vi "Main.vi"(11 "Module Admin":refnum<class "Delacor_lib_QMH_Cloneable Module Admin.lvclass">) -> ()   [LabVIEW 2025, in "USB IO.lvlib"]
doc: "This template is based off of the Queued Message Handler design pattern and the Queued Message Handler project template that ships with LabVIEW.\n\nThe main difference is that the queue is private to this module and communication between modules is performed via Broadcast and Request events.\n\nRequest events are wrapped in public API methods and are handled in the Event Handling Loop (EHL) of this VI. Any module can register for Broadcast events sent by this module. The EHL generates messages based on user interface actions.\n\nThe Message Handling Loop (MHL) processes messages generated by the EHL, or by other messages. The messages are string values, so new messages can be added easily to the Message Cases case structure in the MHL. Each message cluster can also provide an optional value for Message Data, which is a variant that can be converted to whatever message-specific data is required.\n_____\nBased on DQMH Dev Tools: Project Template 7.1.2.1547."
uses:
  USB IO.lvlib
  <vilib>/Delacor/Delacor QMH/Libraries/Message Queue_class/Delacor_lib_QMH_Message Queue.lvclass/Delacor_lib_QMH_Message Queue.ctl
  <vilib>/Delacor/Delacor QMH/Libraries/Cloneable Module Admin_class/Delacor_lib_QMH_Cloneable Module Admin.lvclass/Delacor_lib_QMH_Cloneable Module Admin.ctl
  <vilib>/Delacor/Delacor QMH/Libraries/Module Admin_class/Delacor_lib_QMH_Module Admin.lvclass/Delacor_lib_QMH_Module Admin.ctl
  <vilib>/Delacor/Delacor QMH/Libraries/Message Queue_class/Delacor_lib_QMH_Message Queue.lvclass
  Module Data--cluster.ctl
  <vilib>/Utility/miscctls.llb/LVPointTypeDef.ctl
  <vilib>/Delacor/Delacor QMH/Libraries/Message Queue_class/Delacor_lib_QMH_Enqueue Message (Single).vi
  Stop Argument--cluster.ctl
  <vilib>/Delacor/Delacor QMH/Libraries/Cloneable Module Admin_class/Delacor_lib_QMH_Cloneable Module Admin.lvclass
  Display Lines (Reply Payload)--cluster.ctl
  Display Lines Argument--cluster.ctl
  Classes/USB IO generic/USB IO.lvclass
  select child (Reply Payload)--cluster.ctl
  Classes/Hardware Selection.ctl
  select child Argument--cluster.ctl
  Classes/Arduino Uno/Arduino Uno.lvclass
  Classes/USB-6000/USB-6000.lvclass
  read config (Reply Payload)--cluster.ctl
  read config Argument--cluster.ctl
  init device (Reply Payload)--cluster.ctl
  init device Argument--cluster.ctl
  stop device (Reply Payload)--cluster.ctl
  stop device Argument--cluster.ctl
  C:/Users/grove/Desktop/LabVIEW/Git/dqmh-lvoop-template/Libraries/USB IO/Classes/USB IO generic/USB IO.lvclass
  C:/Users/grove/Desktop/LabVIEW/Git/dqmh-lvoop-template/Libraries/USB IO/Classes/USB-6000/USB-6000.lvclass
  C:/Users/grove/Desktop/LabVIEW/Git/dqmh-lvoop-template/Libraries/USB IO/Classes/Arduino Uno/Arduino Uno.lvclass
panel:
  out "error out":errorcluster
  out "Status":string
  in  "Simulate EHL Error":bool
  in  "Simulate MHL Error":bool
  # "Other processes communicate with this Module via its Public API (wrappers for its Request Events).\n\nThis Module communicates with other processes via its Broadcast Events.\nAny process that wants to receive these messages can register for this module's Broadcast events."
  # "This template is for the DQMH framework. See the block diagram for more information on how to use this template."
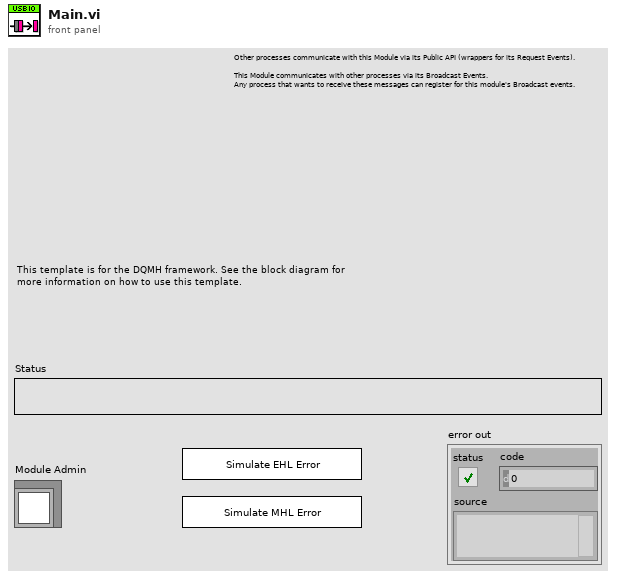
[diagram p1: front panel]
types:
  T1 = typedef "USB IO.lvlib/Request Events--cluster.ctl" = cluster{"Stop Module":refnum<user-event>, "Show Panel":refnum<user-event>, "Hide Panel":refnum<user-event>, "Show Diagram":refnum<user-event>, "Get Module Execution Status":refnum<user-event>, "Display Lines":refnum<user-event>, "select child":refnum<user-event>, "read config":refnum<user-event>, "init":refnum<user-event>, "init device":refnum<user-event>, "stop device":refnum<user-event>}
  T2 = typedef "USB IO.lvlib/Module Data--cluster.ctl" = cluster{"Status":string, "USB IO.lvlib:USB IO.lvclass":refnum<class "USB IO.lvclass">}
  T3 = enum32{"invalid lock state", "Not Locked", "Locked (No Password)", "Password-protected"}
  T4 = typedef "USB IO.lvlib/Stop Argument--cluster.ctl" = cluster{"Module ID":i32, "Origin":string, "Exit via Stop Module Req?":bool, "Wait for Module to stop?":bool}
  T5 = typedef "USB IO.lvlib/Display Lines Argument--cluster.ctl" = cluster{"Module ID":i32, "Wait Notifier":refnum<notifier>, "wait for reply":bool}
  T6 = typedef "USB IO.lvlib/select child Argument--cluster.ctl" = cluster{"Module ID":i32, "Hardware":T7, "Wait Notifier":refnum<notifier>, "wait for reply":bool}
  T7 = typedef "Hardware Selection.ctl" = enum16{"Simulation", "USB-6000", "USB-6001", "Arduino Uno"}
  T8 = typedef "USB IO.lvlib/read config Argument--cluster.ctl" = cluster{"Module ID":i32, "Path":path, "Wait Notifier":refnum<notifier>, "wait for reply":bool}
  T9 = typedef "USB IO.lvlib/init device Argument--cluster.ctl" = cluster{"Module ID":i32, "Variant":variant, "Wait Notifier":refnum<notifier>, "wait for reply":bool}
  T10 = typedef "USB IO.lvlib/stop device Argument--cluster.ctl" = cluster{"Module ID":i32, "Wait Notifier":refnum<notifier>, "wait for reply":bool}
  T11 = typedef "LVPointTypeDef.ctl" = cluster{"Horizontal":i16, "Vertical":i16}
  T12 = enum32{"Invalid", "Standard", "Closed", "Hidden", "Minimized", "Maximized"}
  T13 = typedef "USB IO.lvlib/Display Lines (Reply Payload)--cluster.ctl" = cluster{"Module ID":i32, "Lines":string[], "Values":i32[], "error":errorcluster}
  T14 = typedef "USB IO.lvlib/select child (Reply Payload)--cluster.ctl" = cluster{"Module ID":i32, "error":errorcluster}
  T15 = typedef "USB IO.lvlib/read config (Reply Payload)--cluster.ctl" = cluster{"Module ID":i32, "error":errorcluster}
  T16 = typedef "USB IO.lvlib/init device (Reply Payload)--cluster.ctl" = cluster{"Module ID":i32, "error":errorcluster}
  T17 = typedef "USB IO.lvlib/stop device (Reply Payload)--cluster.ctl" = cluster{"Module ID":i32, "error":errorcluster}
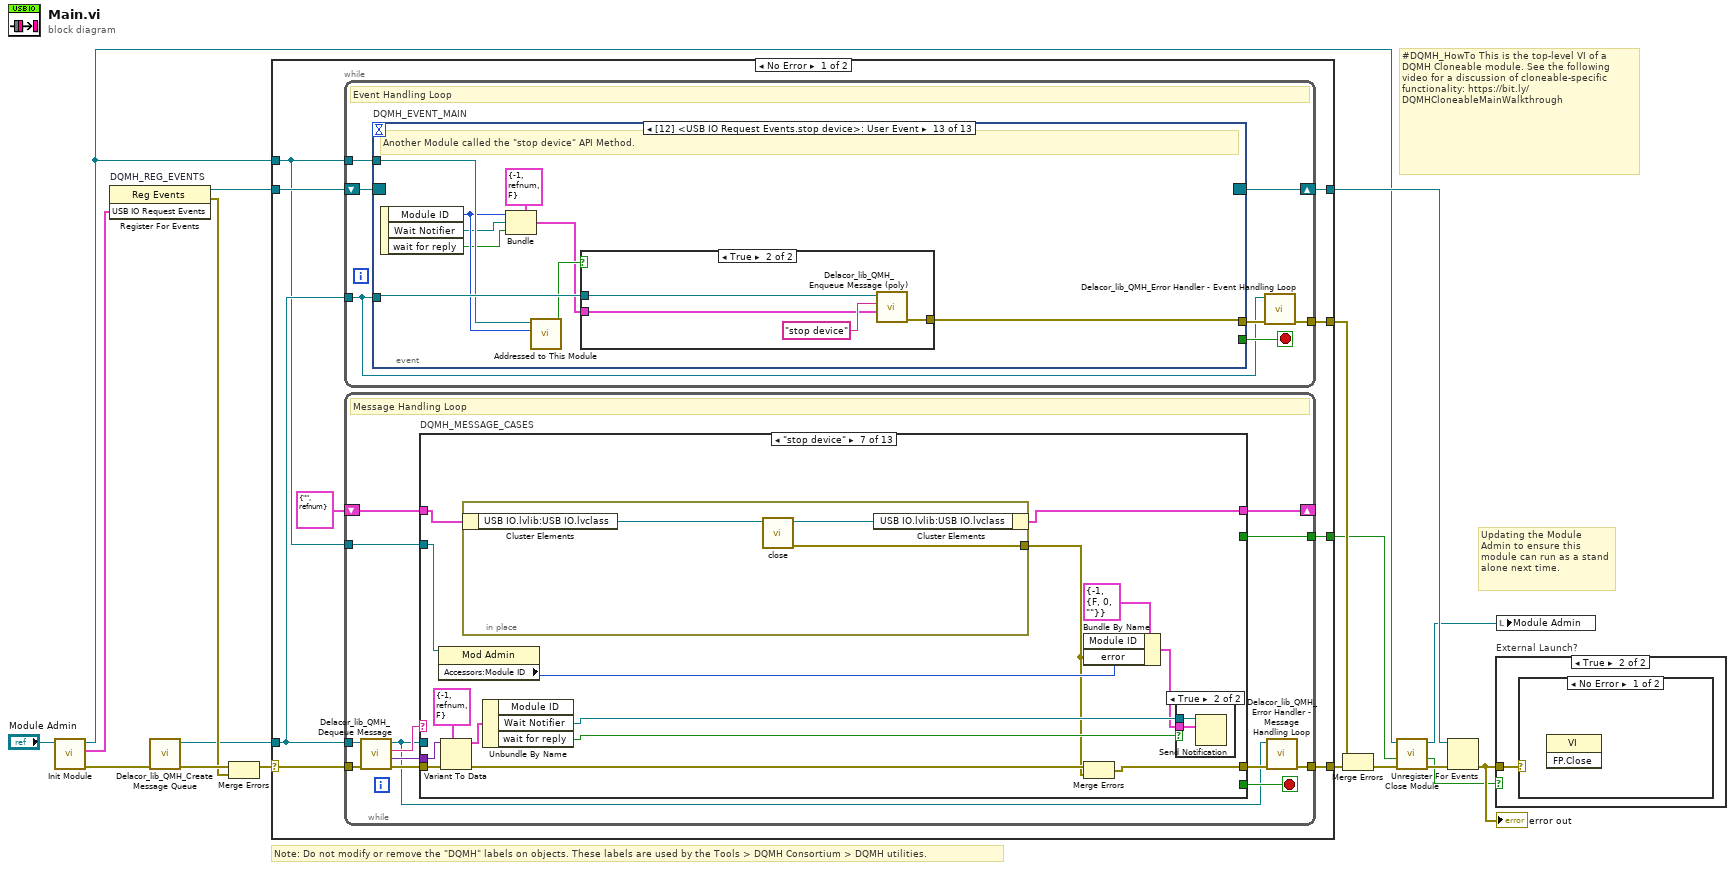
[diagram p0: block diagram]
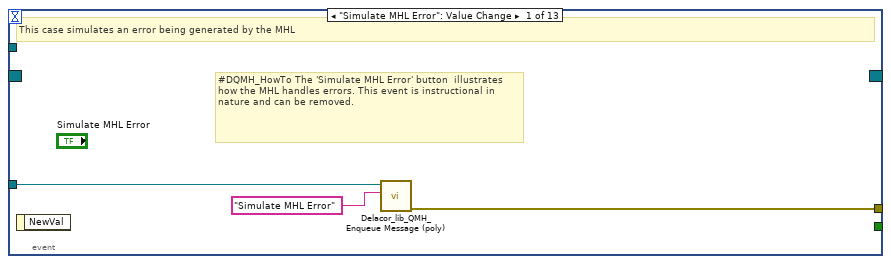
[diagram p2: hidden frame]
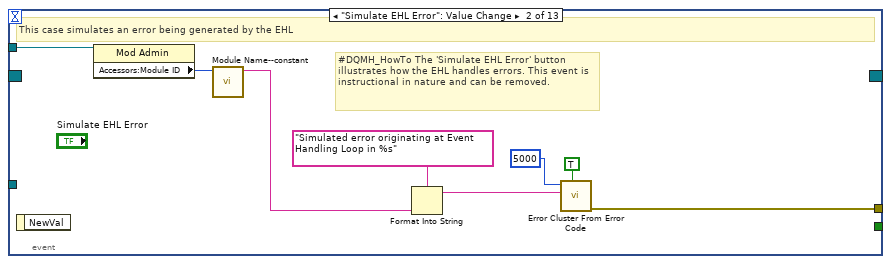
[diagram p3: hidden frame]
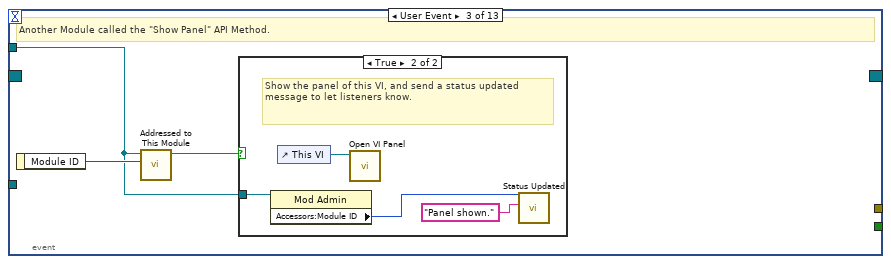
[diagram p4: hidden frame]
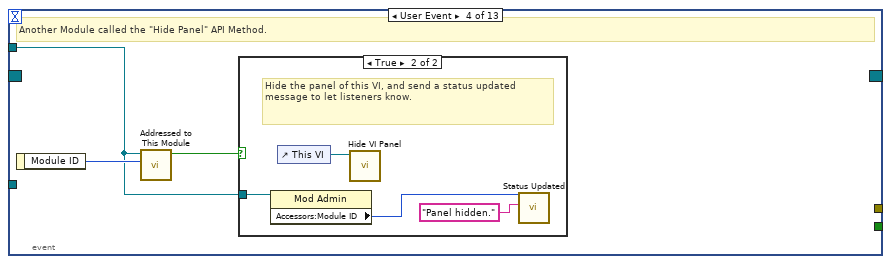
[diagram p6: hidden frame]
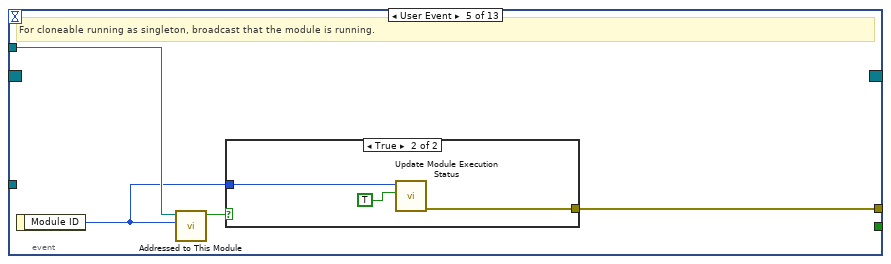
[diagram p8: hidden frame]
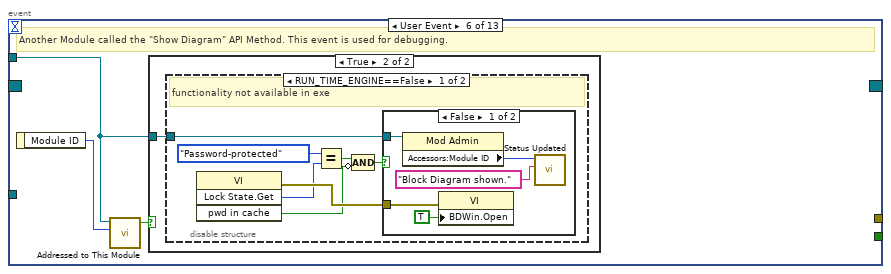
[diagram p10: hidden frame]
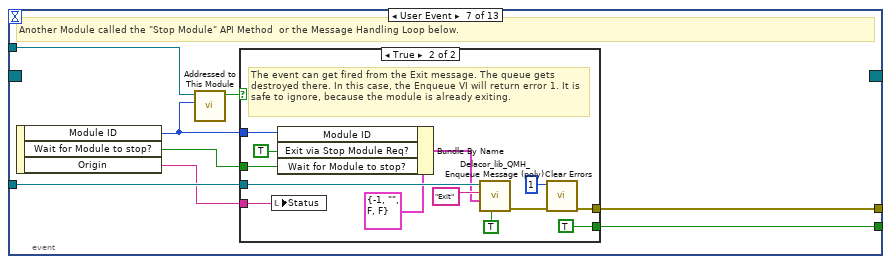
[diagram p14: hidden frame]
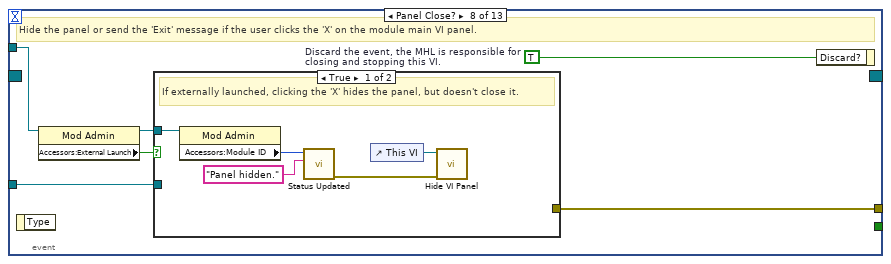
[diagram p16: hidden frame]
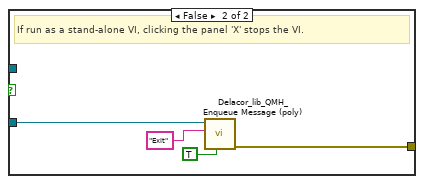
[diagram p17: hidden frame]
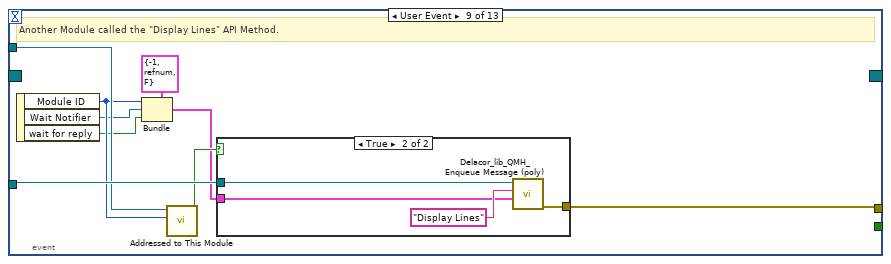
[diagram p18: hidden frame]
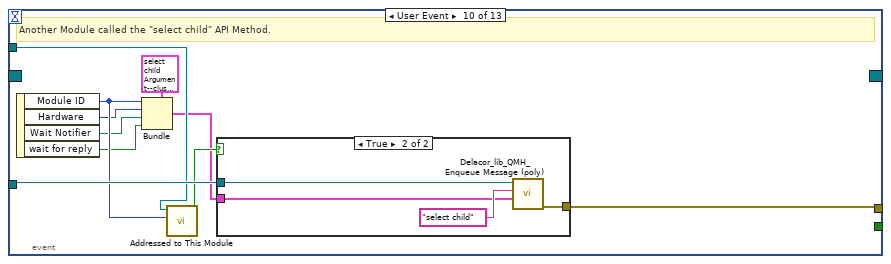
[diagram p20: hidden frame]
diagram:
  # "#DQMH_HowTo This is the top-level VI of a DQMH Cloneable module. See the following video for a discussion of cloneable-specific functionality: https://bit.ly/DQMHCloneableMainWalkthrough"
  # "Note: Do not modify or remove the \"DQMH\" labels on objects. These labels are used by the Tools > DQMH Consortium > DQMH utilities."
  # "Updating the Module Admin to ensure this module can run as a stand alone next time."
  n1 = call "Init Module.vi"("Cloneable Module Admin in"="Module Admin") -> ("error out"=w15:errorcluster, "USB IO Request Events"=w7:T1, "Cloneable Module Admin out"=w4:refnum<class "Delacor_lib_QMH_Cloneable Module Admin.lvclass">)  [unwired: 8 in]
  n2 = register-events "DQMH_REG_EVENTS"(w7) -> (reference out=w8:refnum<event-registration>, error out=w10:errorcluster)  [unwired: 2 in]
  n3 = call <vilib>:"Delacor_lib_QMH_Create Message Queue.vi"("error in"=w15) -> ("error out"=w12:errorcluster, "Message Queue"=w6:refnum<class "Delacor_lib_QMH_Message Queue.lvclass">)  [unwired: 9 in]
  n4 = Merge Errors(w12, w10) -> (w11:errorcluster)
  n5 = case shown="No Error" w11 {
    selector: w11 -> [w25 w404]
    tunnel: [w27 w403] -> w16
    tunnel: [w24 w402] -> w9
    tunnel: w8 -> [w22 w402]
    tunnel: w6 -> [w21 w395]
    tunnel: [w26 _] -> w17
    tunnel: w4 -> [w20 w398]
    tunnel: [w19 _] -> w2
    frame No Error {
      n6 = while {
        tunnel: w21 -> [w28]
        shift-right: [w31] -> w24
        shift-left: w22 -> [w32]
        tunnel: [w33] -> w26
        tunnel: w20 -> [w29]
        stop <- w30 stop-if-true
        # "Event Handling Loop"
        n7 = event "DQMH_EVENT_MAIN" shown="[12] <USB IO Request Events.stop device>: User Event" {
          selector: w32 -> [_ _ _ _ _ _ _ _ _ _ _ _ _]
          dyn-events: [_ _ _ _ _ _ _ _ _ _ _ _ _] -> w31
          timeout: _ -> [_ _ _ _ _ _ _ _ _ _ _ _ _]
          tunnel: [_ _ _ _ _ _ w86 _ _ _ _ _ _] -> w30
          tunnel: w28 -> [w36 _ _ _ _ _ w89 w106 w127 w141 w155 w169 w182]
          tunnel: [w37 w45 _ _ w63 _ w90 w109 w119 w132 w146 w160 w174] -> w34
          tunnel: w29 -> [_ w44 w46 w53 w61 w67 w88 w107 w125 w139 w153 w167 w180]
          event "Simulate MHL Error": Value Change {
            # "#DQMH_HowTo The 'Simulate MHL Error' button  illustrates how the MHL handles errors. This event is instructional in nature and can be removed."
            # "This case simulates an error being generated by the MHL"
            n8 = event-data() -> ()  [unwired: 1 in, 1 out]
            n9 = call-poly <vilib>:"Delacor_lib_QMH_Enqueue Message (poly).vi"("Message"="Simulate MHL Error", "Message Queue in"=w36) -> ("error out"=w37:errorcluster)  [unwired: 8 in, 1 out]
          }
          event "Simulate EHL Error": Value Change {
            # "#DQMH_HowTo The 'Simulate EHL Error' button  illustrates how the EHL handles errors. This event is instructional in nature and can be removed."
            # "This case simulates an error being generated by the EHL"
            n10 = event-data() -> ()  [unwired: 1 in, 1 out]
            n11 = property on="Property Node" class="Mod Admin"(reference=w44) -> ("Accessors:Module ID"=w43:i32)  [unwired: 1 in, 2 out]
            n12 = call "Module Name--constant.vi"("Module ID"=w43) -> ("Module Name"=w38:string)  [unwired: 10 in]
            n13 = Format Into String(format string="Simulated error originating at Event Handling Loop in %s", w38) -> (resulting string=w41:string)  [unwired: 2 in, 1 out]
            n14 = call <vilib>:"Error Cluster From Error Code.vi"("show call chain? (False)"=TRUE, "error message (\"\")"=w41, "error code (0)"=5000) -> ("error out"=w45:errorcluster)  [unwired: 6 in]
          }
          event User Event {
            # "Another Module called the \"Show Panel\" API Method."
            n15 = event-data() -> ("Module ID"=w47:i32)  [unwired: 1 in]
            n16 = call "Addressed to This Module.vi"("Module ID from Argument"=w47, "Module Admin"=w46) -> ("Addressed to this instance?"=w48:bool)  [unwired: 8 in, 1 out]
            n17 = case shown="True" w48 {
              tunnel: w46 -> [_ w50]
              frame False {
              }
              frame True {
                # "Show the panel of this VI, and send a status updated message to let listeners know."
                n18 = property on="Property Node" class="Mod Admin"(reference=w50) -> ("Accessors:Module ID"=w49:i32)  [unwired: 1 in, 2 out]
                n19 = control-ref of="This VI"() -> (w52:refnum<vi>)
                n20 = call "Open VI Panel.vi"("VI"=w52) -> ()  [unwired: 10 in, 1 out]
                n21 = call "Status Updated.vi"("Status"="Panel shown." ("format string"), "Module ID"=w49) -> ()  [unwired: 9 in, 1 out]
              }
            }
          }
          event User Event {
            # "Another Module called the \"Hide Panel\" API Method."
            n22 = event-data() -> ("Module ID"=w54:i32)  [unwired: 1 in]
            n23 = call "Addressed to This Module.vi"("Module ID from Argument"=w54, "Module Admin"=w53) -> ("Addressed to this instance?"=w55:bool)  [unwired: 8 in, 1 out]
            n24 = case shown="True" w55 {
              tunnel: w53 -> [_ w57]
              frame False {
              }
              frame True {
                # "Hide the panel of this VI, and send a status updated message to let listeners know."
                n25 = property on="Property Node" class="Mod Admin"(reference=w57) -> ("Accessors:Module ID"=w56:i32)  [unwired: 1 in, 2 out]
                n26 = control-ref of="This VI"() -> (w59:refnum<vi>)
                n27 = call "Hide VI Panel.vi"("VI"=w59) -> ()  [unwired: 10 in, 1 out]
                n28 = call "Status Updated.vi"("Status"="Panel hidden." ("format string"), "Module ID"=w56) -> ()  [unwired: 9 in, 1 out]
              }
            }
          }
          event User Event {
            # "For cloneable running as singleton, broadcast that the module is running."
            n29 = event-data() -> ("Module ID"=w60:i32)  [unwired: 1 in]
            n30 = call "Addressed to This Module.vi"("Module ID from Argument"=w60, "Module Admin"=w61) -> ("Addressed to this instance?"=w62:bool)  [unwired: 8 in, 1 out]
            n31 = case shown="True" w62 {
              tunnel: [_ w66] -> w63
              tunnel: w60 -> [_ w65]
              frame False {
              }
              frame True {
                n32 = call "Update Module Execution Status.vi"("Running?"=TRUE, "Module ID"=w65) -> ("error out"=w66:errorcluster)  [unwired: 9 in]
              }
            }
          }
          event User Event {
            # "Another Module called the \"Show Diagram\" API Method. This event is used for debugging."
            n33 = event-data() -> ("Module ID"=w68:i32)  [unwired: 1 in]
            n34 = call "Addressed to This Module.vi"("Module ID from Argument"=w68, "Module Admin"=w67) -> ("Addressed to this instance?"=w69:bool)  [unwired: 8 in, 1 out]
            n35 = case shown="True" w69 {
              tunnel: w67 -> [_ w70]
              frame False {
              }
              frame True {
                n36 = disable-structure shown="RUN_TIME_ENGINE==False" {
                  disable-tunnel: w70 -> [w71 _]
                  frame condition #0 (active) {
                    # "functionality not available in exe"
                    n37 = invoke on="Invoke Node" class="VI" method="Lock State.Get"() -> (error out=w77:errorcluster, "Get Lock State"=w76:T3, "pwd in cache"=w73:bool)  [unwired: 4 in, 1 out]
                    n38 = Equal?(x=T3."Password-protected", y=w76) -> (x = y?=w74:bool)
                    n39 = Compound Arithmetic op=AND(w74, invert w73) -> (w72:bool)
                    n40 = case shown="False" w72 {
                      tunnel: w77 -> [w82 _]
                      tunnel: w71 -> [w79 _]
                      frame False {
                        n41 = property on="Property Node" class="Mod Admin"(reference=w79) -> ("Accessors:Module ID"=w78:i32)  [unwired: 1 in, 2 out]
                        n42 = property on="Property Node" class="VI"(error in=w82, "BDWin.Open"=TRUE ("Block Diagram Window:Open")) -> ()  [unwired: 1 in, 2 out]
                        n43 = call "Status Updated.vi"("Status"="Block Diagram shown." ("format string"), "Module ID"=w78) -> ()  [unwired: 9 in, 1 out]
                      }
                      frame True {
                        # "Password-protected VI, and the password is not in the cache. Do not show the diagram."
                      }
                    }
                  }
                  frame condition #1 {
                  }
                }
              }
            }
          }
          event User Event {
            # "Another Module called the \"Stop Module\" API Method  or the Message Handling Loop below."
            n44 = event-data() -> ("Module ID"=w84:i32, "Wait for Module to stop?"=w85:bool, "Origin"=w83:string)  [unwired: 1 in]
            n45 = call "Addressed to This Module.vi"("Module ID from Argument"=w84, "Module Admin"=w88) -> ("Addressed to this instance?"=w87:bool)  [unwired: 8 in, 1 out]
            n46 = case shown="True" w87 {
              tunnel: [_ w102] -> w90
              tunnel: w89 -> [_ w98]
              tunnel: [_ TRUE] -> w86
              tunnel: w85 -> [_ w93]
              tunnel: w84 -> [_ w95]
              tunnel: w83 -> [_ w91]
              frame False {
              }
              frame True {
                # "The event can get fired from the Exit message. The queue gets destroyed there. In this case, the Enqueue VI will return error 1. It is safe to ignore, because the module is already exiting."
                n47 = local write "Status"(w91) -> ()
                n48 = Bundle By Name(cluster=T4 {"Module ID"=-1, "Origin"="", "Exit via Stop Module Req?"=FALSE, "Wait for Module to stop?"=FALSE} ("Stop Argument"), "Module ID"=w95, "Exit via Stop Module Req?"=TRUE, "Wait for Module to stop?"=w93) -> (w92:T4)
                n49 = call-poly <vilib>:"Delacor_lib_QMH_Enqueue Message (poly).vi"("Priority Message? (F)"=TRUE, "Message Data"=w92, "Message"="Exit", "Message Queue in"=w98) -> ("error out"=w103:errorcluster)  [unwired: 6 in, 1 out]
                n50 = call <vilib>:"Clear Errors.vi"("error in (no error)"=w103, "specific error code to clear (0: all)"=1) -> ("error out"=w102:errorcluster)  [unwired: 4 in, 1 out]
              }
            }
          }
          event Panel Close? {
            w108 = TRUE  # Discard the event, the MHL is responsible for closing and stopping this VI.
            # "Hide the panel or send the 'Exit' message if the user clicks the 'X' on the module main VI panel."
            n51 = event-data() -> ()  [unwired: 1 in, 1 out]
            n52 = property on="Property Node" class="Mod Admin"(reference=w107) -> (reference out=w104:refnum<class "Delacor_lib_QMH_Cloneable Module Admin.lvclass">, "Accessors:External Launch"=w105:bool)  [unwired: 1 in, 1 out]
            n53 = case shown="True" w105 {
              tunnel: w106 -> [_ w117]
              tunnel: [_ w118] -> w109
              tunnel: w104 -> [w112 _]
              frame True {
                # "If externally launched, clicking the 'X' hides the panel, but doesn't close it."
                n54 = property on="Property Node" class="Mod Admin"(reference=w112) -> ("Accessors:Module ID"=w111:i32)  [unwired: 1 in, 2 out]
                n55 = call "Status Updated.vi"("Status"="Panel hidden." ("format string"), "Module ID"=w111) -> ("error out"=w110:errorcluster)  [unwired: 9 in]
                n56 = control-ref of="This VI"() -> (w114:refnum<vi>)
                n57 = call "Hide VI Panel.vi"("error in"=w110, "VI"=w114) -> ()  [unwired: 9 in, 1 out]
              }
              frame False {
                # "If run as a stand-alone VI, clicking the panel 'X' stops the VI."
                n58 = call-poly <vilib>:"Delacor_lib_QMH_Enqueue Message (poly).vi"("Priority Message? (F)"=TRUE, "Message"="Exit", "Message Queue in"=w117) -> ("error out"=w118:errorcluster)  [unwired: 7 in, 1 out]
              }
            }
            n59 = event-data ("Event Filter Node")("Discard?"=w108) -> ()  [unwired: 1 in, 1 out]
          }
          event User Event {
            # "Another Module called the \"Display Lines\" API Method."
            n60 = event-data() -> ("Module ID"=w122:i32, "Wait Notifier"=w121:refnum<notifier>, "wait for reply"=w120:bool)  [unwired: 1 in]
            n61 = Bundle(cluster=T5 {"Module ID"=-1, "Wait Notifier"=refnum, "wait for reply"=FALSE} ("Display Lines Argument"), "Module ID"=w122, "Wait Notifier"=w121, "wait for reply"=w120) -> (w123:T5)
            n62 = call "Addressed to This Module.vi"("Module ID from Argument"=w122, "Module Admin"=w125) -> ("Addressed to this instance?"=w126:bool)  [unwired: 8 in, 1 out]
            n63 = case shown="True" w126 {
              tunnel: w127 -> [_ w131]
              tunnel: w123 -> [_ w129]
              tunnel: [_ w128] -> w119
              frame False {
              }
              frame True {
                n64 = call-poly <vilib>:"Delacor_lib_QMH_Enqueue Message (poly).vi"("Message Data"=w129, "Message"="Display Lines", "Message Queue in"=w131) -> ("error out"=w128:errorcluster)  [unwired: 7 in, 1 out]
              }
            }
          }
          event User Event {
            # "Another Module called the \"select child\" API Method."
            n65 = event-data() -> ("Module ID"=w136:i32, "Hardware"=w135:T7, "Wait Notifier"=w134:refnum<notifier>, "wait for reply"=w133:bool)  [unwired: 1 in]
            n66 = Bundle(cluster=T6 {"Module ID"=-1, "Hardware"=enum."USB-6000", "Wait Notifier"=refnum, "wait for reply"=FALSE} ("select child Argument"), "Module ID"=w136, "Hardware"=w135, "Wait Notifier"=w134, "wait for reply"=w133) -> (w137:T6)
            n67 = call "Addressed to This Module.vi"("Module ID from Argument"=w136, "Module Admin"=w139) -> ("Addressed to this instance?"=w140:bool)  [unwired: 8 in, 1 out]
            n68 = case shown="True" w140 {
              tunnel: w141 -> [_ w145]
              tunnel: w137 -> [_ w143]
              tunnel: [_ w142] -> w132
              frame False {
              }
              frame True {
                n69 = call-poly <vilib>:"Delacor_lib_QMH_Enqueue Message (poly).vi"("Message Data"=w143, "Message"="select child", "Message Queue in"=w145) -> ("error out"=w142:errorcluster)  [unwired: 7 in, 1 out]
              }
            }
          }
          event User Event {
            # "Another Module called the \"read config\" API Method."
            n70 = event-data() -> ("Module ID"=w150:i32, "Path"=w149:path, "Wait Notifier"=w148:refnum<notifier>, "wait for reply"=w147:bool)  [unwired: 1 in]
            n71 = Bundle(cluster=T8 {"Module ID"=-1, "Path"=path "", "Wait Notifier"=refnum, "wait for reply"=FALSE} ("read config Argument"), "Module ID"=w150, "Path"=w149, "Wait Notifier"=w148, "wait for reply"=w147) -> (w151:T8)
            n72 = call "Addressed to This Module.vi"("Module ID from Argument"=w150, "Module Admin"=w153) -> ("Addressed to this instance?"=w154:bool)  [unwired: 8 in, 1 out]
            n73 = case shown="True" w154 {
              tunnel: w155 -> [_ w159]
              tunnel: w151 -> [_ w157]
              tunnel: [_ w156] -> w146
              frame False {
              }
              frame True {
                n74 = call-poly <vilib>:"Delacor_lib_QMH_Enqueue Message (poly).vi"("Message Data"=w157, "Message"="read config", "Message Queue in"=w159) -> ("error out"=w156:errorcluster)  [unwired: 7 in, 1 out]
              }
            }
          }
          event User Event {
            # "Another Module called the \"init device\" API Method."
            n75 = event-data() -> ("Module ID"=w164:i32, "Variant"=w163:variant, "Wait Notifier"=w162:refnum<notifier>, "wait for reply"=w161:bool)  [unwired: 1 in]
            n76 = Bundle(cluster=T9 {"Module ID"=-1, "Variant"=variant, "Wait Notifier"=refnum, "wait for reply"=FALSE} ("init device Argument"), "Module ID"=w164, "Variant"=w163, "Wait Notifier"=w162, "wait for reply"=w161) -> (w165:T9)
            n77 = call "Addressed to This Module.vi"("Module ID from Argument"=w164, "Module Admin"=w167) -> ("Addressed to this instance?"=w168:bool)  [unwired: 8 in, 1 out]
            n78 = case shown="True" w168 {
              tunnel: w169 -> [_ w173]
              tunnel: w165 -> [_ w171]
              tunnel: [_ w170] -> w160
              frame False {
              }
              frame True {
                n79 = call-poly <vilib>:"Delacor_lib_QMH_Enqueue Message (poly).vi"("Message Data"=w171, "Message"="init device", "Message Queue in"=w173) -> ("error out"=w170:errorcluster)  [unwired: 7 in, 1 out]
              }
            }
          }
          event User Event {
            # "Another Module called the \"stop device\" API Method."
            n80 = event-data() -> ("Module ID"=w177:i32, "Wait Notifier"=w176:refnum<notifier>, "wait for reply"=w175:bool)  [unwired: 1 in]
            n81 = Bundle(cluster=T10 {"Module ID"=-1, "Wait Notifier"=refnum, "wait for reply"=FALSE} ("stop device Argument"), "Module ID"=w177, "Wait Notifier"=w176, "wait for reply"=w175) -> (w178:T10)
            n82 = call "Addressed to This Module.vi"("Module ID from Argument"=w177, "Module Admin"=w180) -> ("Addressed to this instance?"=w181:bool)  [unwired: 8 in, 1 out]
            n83 = case shown="True" w181 {
              tunnel: w182 -> [_ w186]
              tunnel: w178 -> [_ w184]
              tunnel: [_ w183] -> w174
              frame False {
              }
              frame True {
                n84 = call-poly <vilib>:"Delacor_lib_QMH_Enqueue Message (poly).vi"("Message Data"=w184, "Message"="stop device", "Message Queue in"=w186) -> ("error out"=w183:errorcluster)  [unwired: 7 in, 1 out]
              }
            }
          }
        }
        n85 = call-dynamic "Delacor_lib_QMH_Error Handler - Event Handling Loop.vi"("error in"=w34, "Message Queue in"=w28) -> ("dup error in"=w33:errorcluster)  [unwired: 8 in, 1 out]
      }
      n86 = while {
        tunnel: w21 -> [w187]
        shift-right: [w194] -> _
        shift-left: T2 {"Status"="", "USB IO.lvlib:USB IO.lvclass"=refnum} ("Data Cluster") -> [w195]
        tunnel: w25 -> [w198]
        tunnel: [w196] -> w27
        tunnel: w20 -> [w189]
        tunnel: [w188] -> w19
        stop <- w193 stop-if-true
        # "Message Handling Loop"
        n87 = call-dynamic "Delacor_lib_QMH_Dequeue Message.vi"("error in"=w198, "Message Queue in"=w187) -> ("error out"=w197:errorcluster, "Message Data"=w191:variant, "Message"=w192:string, "Message Queue out"=w190:refnum<class "Delacor_lib_QMH_Message Queue.lvclass">)  [unwired: 6 in]
        n88 = case "DQMH_MESSAGE_CASES" shown="\"stop device\"" w192 {
          selector: w192 -> [_ _ _ _ _ _ _ _ _ _ _ _ w384]
          tunnel: w190 -> [_ _ _ _ _ _ _ _ _ w339 _ w376 _]
          tunnel: w197 -> [w218 w222 w239 w262 w284 w306 w326 w334 w336 w348 w365 w382 w393]
          tunnel: [w216 w222 w230 w253 w275 w297 w317 w333 w336 w344 w364 w377 w394] -> w199
          tunnel: w195 -> [w209 w221 w226 w250 w272 w294 w314 w332 w335 w343 w362 w375 w391]
          tunnel: [w208 w221 w227 w248 w271 w293 w313 w332 w335 w343 w362 w375 w391] -> w194
          tunnel: [_ _ _ _ _ _ _ _ _ _ _ w374 _] -> w193
          tunnel: w191 -> [_ _ w237 w260 w282 w304 w324 _ _ w342 _ w372 _]
          tunnel: w189 -> [w204 _ w228 w251 w273 w295 w315 _ _ w341 w360 w367 w390]
          tunnel: [_ _ _ _ _ _ _ _ _ _ _ w370 _] -> w188
          frame "Initialize" {
            w201 = "Initial Message" ("Initial Message")
            # "#DQMH_CodeNeeded - Initialize the appearance of the front panel."
            # "#DQMH_CodeNeeded - Initialize your state data here."
            # "Initialize - Any operation that needs to be done before the module can receive messages. Synchronize Caller Events.vi will inform Start Module.vi that the module has launched and is ready to receive messages. Module Did Init.vi will broadcast that the module initialized."
            n89 = call "Synchronize Caller Events.vi"("error in"=w218, "Module Admin"=w204) -> ("error out"=w217:errorcluster, "Module Admin out"=w203:refnum<class "Delacor_lib_QMH_Cloneable Module Admin.lvclass">)  [unwired: 8 in]
            n90 = property on="Property Node" class="Mod Admin"(reference=w203) -> ("Accessors:Module ID"=w200:i32, "Accessors:External Launch"=w205:bool)  [unwired: 1 in, 2 out]
            n91 = call "Module Name--constant.vi"("Module ID"=w200) -> ("Module Name"=w213:string)  [unwired: 10 in]
            n92 = property on="Property Node" class="VI"("Front Panel.Title"=w213) -> (reference out=w215:refnum<vi>, error out=w220:errorcluster)  [unwired: 2 in]
            n93 = Select(t=T12."Hidden" ("State"), s=w205, f=T12."Standard" ("State")) -> (s? t:f=w210:T12)
            n94 = invoke on="Invoke Node" class="VI" method="FP.Open"(reference=w215, error in=w220, "State"=w210) -> (reference out=w214:refnum<vi>, error out=w219:errorcluster)  [unwired: 2 in, 3 out]
            n95 = Bundle By Name(cluster=w209, "Status"=w201) -> (w208:T2)
            n96 = invoke on="Invoke Node" class="VI" method="FP.Center"(reference=w214, error in=w219) -> ()  [unwired: 1 in, 3 out]
            n97 = property on="Pane" class="Pane"("Origin"=T11 {"Horizontal"=0, "Vertical"=0}) -> ()  [unwired: 2 in, 2 out]
            n98 = call "Module Name--constant.vi"("Module ID"=w200) -> ("Module Name"=w206:string)  [unwired: 10 in]
            n99 = call "Module Did Init.vi"("error in"=w217, "Initialized?"=TRUE, "Origin"=w206, "Module ID"=w200) -> ("error out"=w216:errorcluster)  [unwired: 7 in]
            "Status" <- w201
          }
          frame "---Module Specific---" {
            # "Separator -- The following cases handle messages specific to this Module."
          }
          frame "Display Lines" {
            n100 = property class="Mod Admin"(reference=w228) -> ("Accessors:Module ID"=w229:i32)  [unwired: 1 in, 2 out]
            n101 = Variant To Data(error in=w239, type=T5 {"Module ID"=-1, "Wait Notifier"=refnum, "wait for reply"=FALSE} ("Display Lines Argument"), Variant=w237) -> (data=w235:T5, error out=w238:errorcluster)
            n102 = in-place {
              in-place-border: [w242] -> w225
              in-place-border: [w241] -> w224
              in-place-border: [w240] -> w223
              n103 = in-place-cluster #1(w226) -> ("USB IO.lvlib:USB IO.lvclass"=w244:refnum<class "USB IO.lvclass">)
              n104 = call-dynamic "display lines.vi"("USB IO in"=w244) -> ("error out"=w240:errorcluster, "Values"=w241:i32[], "Lines"=w242:string[], "USB IO out"=w243:refnum<class "USB IO.lvclass">)  [unwired: 7 in]
              n105 = in-place-cluster #1("USB IO.lvlib:USB IO.lvclass"=w243) -> (w227:T2)
            }
            n106 = Unbundle By Name(w235) -> ("Wait Notifier"=w234:refnum<notifier>, "wait for reply"=w233:bool)  [unwired: 1 out]
            n107 = Bundle By Name(cluster=T13 {"Module ID"=-1, "Lines"=[], "Values"=[], "error"={"status"=FALSE, "code"=0, "source"=""}} ("Display Lines (Reply Payload)"), "Module ID"=w229, "Lines"=w225, "Values"=w224, "error"=w223) -> (w232:T13)
            n108 = Merge Errors(w238, w223) -> (w230:errorcluster)
            n109 = case "DQMH_FIRE_NOTIFIER" shown="True" w233 {
              tunnel: w234 -> [_ w246]
              tunnel: w232 -> [_ w245]
              frame False {
              }
              frame True {
                n110 = Send Notification(notification=w245, notifier=w246) -> ()  [unwired: 1 in, 2 out]
              }
            }
          }
          frame "select child" {
            w247 = errorcluster {"status"=FALSE, "code"=0, "source"=""} ("error")
            n111 = property class="Mod Admin"(reference=w251) -> ("Accessors:Module ID"=w252:i32)  [unwired: 1 in, 2 out]
            n112 = Variant To Data(error in=w262, type=T6 {"Module ID"=-1, "Hardware"=enum."USB-6000", "Wait Notifier"=refnum, "wait for reply"=FALSE} ("select child Argument"), Variant=w260) -> (data=w258:T6, error out=w261:errorcluster)
            n113 = Unbundle By Name(w258) -> ("Hardware"=w249:T7, "Wait Notifier"=w257:refnum<notifier>, "wait for reply"=w256:bool)  [unwired: 1 out]
            n114 = in-place {
              in-place-border: w249 -> [w264]
              n115 = in-place-cluster #2(w250) -> ()  [unwired: 1 out]
              n116 = case shown="\"USB-6000\", Default" w264 {
                tunnel: [refnum<class "USB-6000.lvclass"> refnum ("USB IO.lvlib:USB-6000.lvclass") refnum<class "Arduino Uno.lvclass"> refnum ("USB IO.lvlib:Arduino Uno.lvclass")] -> w263
                frame "USB-6000", Default {
                }
                frame "Arduino Uno" {
                }
              }
              n117 = in-place-cluster #2("USB IO.lvlib:USB IO.lvclass"=w263) -> (w248:T2)
            }
            n118 = Bundle By Name(cluster=T14 {"Module ID"=-1, "error"={"status"=FALSE, "code"=0, "source"=""}} ("select child (Reply Payload)"), "Module ID"=w252, "error"=w247) -> (w255:T14)
            n119 = Merge Errors(w261, w247) -> (w253:errorcluster)
            n120 = case "DQMH_FIRE_NOTIFIER" shown="True" w256 {
              tunnel: w257 -> [_ w268]
              tunnel: w255 -> [_ w267]
              frame False {
              }
              frame True {
                n121 = Send Notification(notification=w267, notifier=w268) -> ()  [unwired: 1 in, 2 out]
              }
            }
          }
          frame "read config" {
            n122 = property class="Mod Admin"(reference=w273) -> ("Accessors:Module ID"=w274:i32)  [unwired: 1 in, 2 out]
            n123 = Variant To Data(error in=w284, type=T8 {"Module ID"=-1, "Path"=path "", "Wait Notifier"=refnum, "wait for reply"=FALSE} ("read config Argument"), Variant=w282) -> (data=w280:T8, error out=w283:errorcluster)
            n124 = Unbundle By Name(w280) -> ("Path"=w270:path, "Wait Notifier"=w279:refnum<notifier>, "wait for reply"=w278:bool)  [unwired: 1 out]
            n125 = in-place {
              in-place-border: w270 -> [w286]
              in-place-border: [w285] -> w269
              n126 = in-place-cluster #3(w272) -> ("USB IO.lvlib:USB IO.lvclass"=w288:refnum<class "USB IO.lvclass">)
              n127 = call-dynamic "read config.vi"("Path"=w286, "USB IO in"=w288) -> ("error out"=w285:errorcluster, "USB IO out"=w287:refnum<class "USB IO.lvclass">)  [unwired: 8 in]
              n128 = in-place-cluster #3("USB IO.lvlib:USB IO.lvclass"=w287) -> (w271:T2)
            }
            n129 = Bundle By Name(cluster=T15 {"Module ID"=-1, "error"={"status"=FALSE, "code"=0, "source"=""}} ("read config (Reply Payload)"), "Module ID"=w274, "error"=w269) -> (w277:T15)
            n130 = Merge Errors(w283, w269) -> (w275:errorcluster)
            n131 = case "DQMH_FIRE_NOTIFIER" shown="True" w278 {
              tunnel: w279 -> [_ w290]
              tunnel: w277 -> [_ w289]
              frame False {
              }
              frame True {
                n132 = Send Notification(notification=w289, notifier=w290) -> ()  [unwired: 1 in, 2 out]
              }
            }
          }
          frame "init device" {
            n133 = property class="Mod Admin"(reference=w295) -> ("Accessors:Module ID"=w296:i32)  [unwired: 1 in, 2 out]
            n134 = Variant To Data(error in=w306, type=T9 {"Module ID"=-1, "Variant"=variant, "Wait Notifier"=refnum, "wait for reply"=FALSE} ("init device Argument"), Variant=w304) -> (data=w302:T9, error out=w305:errorcluster)
            n135 = Unbundle By Name(w302) -> ("Variant"=w291:variant, "Wait Notifier"=w301:refnum<notifier>, "wait for reply"=w300:bool)  [unwired: 1 out]
            n136 = in-place {
              in-place-border: [w307] -> w292
              in-place-border: w291 -> [_]
              n137 = in-place-cluster #4(w294) -> ("USB IO.lvlib:USB IO.lvclass"=w309:refnum<class "USB IO.lvclass">)
              n138 = call-dynamic "init.vi"("USB IO in"=w309) -> ("error out"=w307:errorcluster, "USB IO out"=w308:refnum<class "USB IO.lvclass">)  [unwired: 9 in]
              n139 = in-place-cluster #4("USB IO.lvlib:USB IO.lvclass"=w308) -> (w293:T2)
            }
            n140 = Bundle By Name(cluster=T16 {"Module ID"=-1, "error"={"status"=FALSE, "code"=0, "source"=""}} ("init device (Reply Payload)"), "Module ID"=w296, "error"=w292) -> (w299:T16)
            n141 = Merge Errors(w305, w292) -> (w297:errorcluster)
            n142 = case "DQMH_FIRE_NOTIFIER" shown="True" w300 {
              tunnel: w301 -> [_ w311]
              tunnel: w299 -> [_ w310]
              frame False {
              }
              frame True {
                n143 = Send Notification(notification=w310, notifier=w311) -> ()  [unwired: 1 in, 2 out]
              }
            }
          }
          frame "stop device" {
            n144 = property class="Mod Admin"(reference=w315) -> ("Accessors:Module ID"=w316:i32)  [unwired: 1 in, 2 out]
            n145 = Variant To Data(error in=w326, type=T10 {"Module ID"=-1, "Wait Notifier"=refnum, "wait for reply"=FALSE} ("stop device Argument"), Variant=w324) -> (data=w322:T10, error out=w325:errorcluster)
            n146 = in-place {
              in-place-border: [w327] -> w312
              n147 = in-place-cluster #5(w314) -> ("USB IO.lvlib:USB IO.lvclass"=w329:refnum<class "USB IO.lvclass">)
              n148 = call-dynamic "close.vi"("USB IO in"=w329) -> ("error out"=w327:errorcluster, "USB IO out"=w328:refnum<class "USB IO.lvclass">)  [unwired: 9 in]
              n149 = in-place-cluster #5("USB IO.lvlib:USB IO.lvclass"=w328) -> (w313:T2)
            }
            n150 = Unbundle By Name(w322) -> ("Wait Notifier"=w321:refnum<notifier>, "wait for reply"=w320:bool)  [unwired: 1 out]
            n151 = Bundle By Name(cluster=T17 {"Module ID"=-1, "error"={"status"=FALSE, "code"=0, "source"=""}} ("stop device (Reply Payload)"), "Module ID"=w316, "error"=w312) -> (w319:T17)
            n152 = Merge Errors(w325, w312) -> (w317:errorcluster)
            n153 = case "DQMH_FIRE_NOTIFIER" shown="True" w320 {
              tunnel: w321 -> [_ w331]
              tunnel: w319 -> [_ w330]
              frame False {
              }
              frame True {
                n154 = Send Notification(notification=w330, notifier=w331) -> ()  [unwired: 1 in, 2 out]
              }
            }
          }
          frame "---Copy This Frame---" {
            # "Duplicate this frame when creating new messages.  Change this comment in the duplicated frame to describe this message."
            n155 = Merge Errors(w334) -> (w333:errorcluster)
          }
          frame "---Exit and Error Handling---" {
            # "Separator - the following cases handle errors and exit messages."
          }
          frame "Error" {
            # "#DQMH_CodeRecommended - If the module is running in standalone mode (External Launch = FALSE), this code will pop up an error dialog and call the 'Exit' message if an error occurs. Add more fine-grained error management here."
            # "Error - Check the error message data and respond accordingly. This message is sent by the \"Error Handler\" VIs at the end of each loop in this application."
            n156 = property on="Property Node" class="Mod Admin"(reference=w341) -> ("Accessors:External Launch"=w340:bool, "Accessors:Module ID"=w338:i32)  [unwired: 1 in, 2 out]
            n157 = Variant To Data(error in=w348, type=errorcluster {"status"=FALSE, "code"=0, "source"=""} ("error constant"), Variant=w342) -> (data=w337:errorcluster, error out=w346:errorcluster)
            n158 = local write "error out"(w337) -> ()
            n159 = call "Error Reported.vi"("Error"=w337, "Module ID"=w338) -> ()  [unwired: 9 in, 1 out]
            n160 = case shown="False" w340 {
              tunnel: [w353 _] -> w345
              tunnel: w339 -> [w351 _]
              tunnel: w337 -> [w352 _]
              frame False {
                n161 = disable-structure shown="Default" {
                  disable-tunnel: w352 -> [w354 _]
                  frame condition #0 (active) {
                    # "If the module is running standalone, then pop up an error dialog and call the \"Exit\" message."
                    n162 = call <vilib>:"Simple Error Handler.vi"("error in (no error)"=w354) -> ()  [unwired: 4 in, 5 out]
                  }
                  frame condition #1 {
                    # "To prevent the Simple Error Handler VI from being loaded (e.g. when deploying to a Real-Time target), add the Conditional Disable Symbol \"DQMH_Disable_SEH\" to your project and set it to TRUE."
                  }
                }
                n163 = call-poly <vilib>:"Delacor_lib_QMH_Enqueue Message (poly).vi"("Priority Message? (F)"=TRUE, "Message"="Exit", "Message Queue in"=w351) -> ("error out"=w353:errorcluster)  [unwired: 7 in, 1 out]
              }
              frame True {
                # "If the module was launched externally, calling the Error Reported broadcast VI is the only action performed by the \"Error\" message. The module's caller can then process the error appropriately."
              }
            }
            n164 = Merge Errors(w346, w345) -> (w344:errorcluster)
          }
          frame "Simulate MHL Error" {
            # "#DQMH_HowTo The 'Simulate MHL Error' button  illustrates how the MHL handles errors. This event is instructional in nature and can be removed."
            # "Simulate an error occurring at the MHL"
            n165 = property on="Property Node" class="Mod Admin"(reference=w360) -> ("Accessors:Module ID"=w361:i32)  [unwired: 1 in, 2 out]
            n166 = call "Module Name--constant.vi"("Module ID"=w361) -> ("Module Name"=w356:string)  [unwired: 10 in]
            n167 = Format Into String(format string="Simulated error originating at Message Handling Loop in %s", w356) -> (resulting string=w357:string)  [unwired: 2 in, 1 out]
            n168 = call <vilib>:"Error Cluster From Error Code.vi"("show call chain? (False)"=TRUE, "error message (\"\")"=w357, "error code (0)"=5001) -> ("error out"=w363:errorcluster)  [unwired: 6 in]
            n169 = Merge Errors(w365, w363) -> (w364:errorcluster)
          }
          frame "Exit" {
            w373 = 91  # 91: not all Exit messages will have an argument
            w374 = TRUE  # Stop the VI
            # "Release the message queue reference"
            # "#DQMH_CodeNeeded - Add any required cleanup code here."
            # "Exit - Exit the application."
            n170 = Variant To Data(error in=w382, type=T4 {"Module ID"=-1, "Origin"="", "Exit via Stop Module Req?"=FALSE, "Wait for Module to stop?"=FALSE} ("Stop Argument"), Variant=w372) -> (data=w369:T4, error out=w378:errorcluster)
            n171 = call <vilib>:"Clear Errors.vi"("error in (no error)"=w378, "specific error code to clear (0: all)"=w373) -> ("error out"=w381:errorcluster)  [unwired: 4 in, 1 out]
            n172 = property on="Property Node" class="Mod Admin"(reference=w367) -> ("Accessors:Module ID"=w366:i32)  [unwired: 1 in, 2 out]
            n173 = control-ref of="This VI"() -> (w368:refnum<vi>)
            n174 = call-dynamic "Delacor_lib_QMH_Release Message Queue.vi"("error in"=w381, "Message Queue"=w376) -> ("error out"=w380:errorcluster)  [unwired: 9 in]
            n175 = call "Handle Exit.vi"("Stop Argument"=w369, "Module Admin in"=w367, "VI reference"=w368) -> ("error out"=w379:errorcluster, "Wait for Stop?"=w370:bool)  [unwired: 7 in]
            n176 = Merge Errors(w380, w379) -> (w377:errorcluster)
            n177 = call "Error Reported.vi"("Error"=w377, "Module ID"=w366) -> ()  [unwired: 9 in, 1 out]
          }
          frame Default {
            # "'Default' case only runs if there is a message that isn't defined in any of the other cases.  Output a programming error."
            n178 = property on="Property Node" class="Mod Admin"(reference=w390) -> ("Accessors:Module ID"=w389:i32)  [unwired: 1 in, 2 out]
            n179 = call "Module Name--constant.vi"("Module ID"=w389) -> ("Module Name"=w383:string)  [unwired: 10 in]
            n180 = Format Into String(format string="The invalid message string \"%s\" was received in the Message Handling Loop for module \"%s\".", w384, w383) -> (resulting string=w386:string)  [unwired: 2 in, 1 out]
            n181 = call <vilib>:"Error Cluster From Error Code.vi"("show call chain? (False)"=TRUE, "error message (\"\")"=w386, "error code (0)"=1) -> ("error out"=w392:errorcluster)  [unwired: 6 in]
            n182 = Merge Errors(w393, w392) -> (w394:errorcluster)
          }
        }
        n183 = call-dynamic "Delacor_lib_QMH_Error Handler - Message Handling Loop.vi"("error in"=w199, "Message Queue in"=w190) -> ("dup error in"=w196:errorcluster)  [unwired: 8 in, 1 out]
      }
    }
    frame Error {
      n184 = call "Synchronize Caller Events.vi"("Module Admin"=w398) -> ("Module Admin out"=w397:refnum<class "Delacor_lib_QMH_Cloneable Module Admin.lvclass">)  [unwired: 9 in, 1 out]
      n185 = property on="Property Node" class="Mod Admin"(reference=w397) -> ("Accessors:Module ID"=w396:i32)  [unwired: 1 in, 2 out]
      n186 = call-dynamic "Delacor_lib_QMH_Release Message Queue.vi"("error in"=w404, "Message Queue"=w395) -> ("error out"=w403:errorcluster)  [unwired: 9 in]
      n187 = call "Module Name--constant.vi"("Module ID"=w396) -> ("Module Name"=w401:string)  [unwired: 10 in]
      n188 = Format Into String(format string="An error occurred during initialization. %s is no longer running.", w401) -> (resulting string=w399:string)  [unwired: 2 in, 1 out]
      n189 = call "Error Reported.vi"("Additional Information"=w399, "Error"=w403, "Module ID"=w396) -> ()  [unwired: 8 in, 1 out]
    }
  }
  n190 = Merge Errors(w17, w16) -> (w18:errorcluster)
  n191 = call "Close Module.vi"("error in"=w18, "Wait for stop?"=w2, "Module Admin in"=w4) -> ("error out"=w14:errorcluster, "External Launch"=w1:bool, "Module Admin out"=w3:refnum<class "Delacor_lib_QMH_Cloneable Module Admin.lvclass">)  [unwired: 6 in]
  n192 = Unregister For Events(event registration refnum=w9, error in=w14) -> (error out=w13:errorcluster)
  "error out" <- w13
  n193 = case "External Launch?" shown="True" w1 {
    tunnel: w13 -> [_ w405]
    frame False {
    }
    frame True {
      n194 = case shown="No Error" w405 {
        frame No Error {
          n195 = invoke class="VI" method="FP.Close"() -> ()  [unwired: 3 in, 3 out]
        }
        frame Error {
          n196 = disable-structure shown="Default" {
            frame condition #0 (active) {
              n197 = invoke class="VI" method="FP.Open"("Activate"=TRUE ("Activate?")) -> ()  [unwired: 4 in, 5 out]
            }
            frame condition #1 {
              # "Don't show panel on error if running inside a built EXE."
            }
          }
        }
      }
    }
  }
  n198 = local write "Module Admin"(w3) -> ()
